vi "absolute_position.vi"(6 "ENCODER rotates cw":bool, 7 "curr. angle":dbl format="%#_13g", 8 "Absolute position in":dbl=-1.0, 11 "prev. angle":dbl format="%#_13g") -> (0 "Absolute position out":dbl, 1 "relative position Gantry":dbl, 2 "relative position shaft":dbl, 3 "Gantry Position (abs)":dbl)   [LabVIEW 2021]
panel:
  out "abs(x)":dbl
  out "angular step > 8deg and <345?":bool
  out "angular difference":dbl
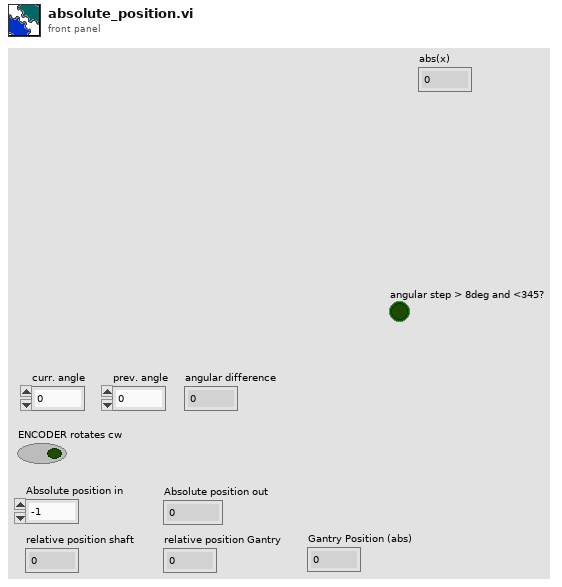
[diagram p1: front panel]
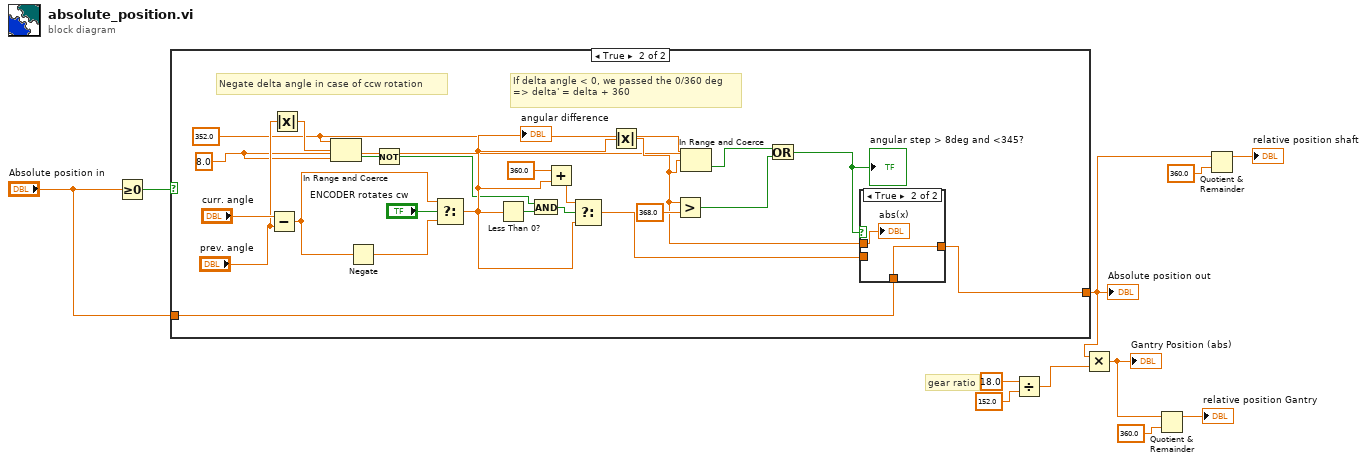
[diagram p0: block diagram]
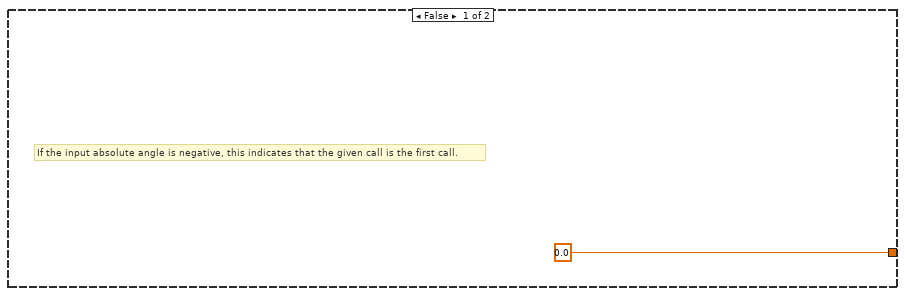
[diagram p2: hidden frame]
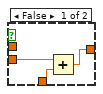
[diagram p3: hidden frame]
diagram:
  # "gear ratio"
  n1 = Greater Or Equal To 0?(x="Absolute position in") -> (x >= 0?=w8:bool)
  n2 = case shown="True" w8 {
    tunnel: "Absolute position in" -> [_ w29]
    tunnel: [0.0 w27] -> w5
    frame False {
      # "If the input absolute angle is negative, this indicates that the given call is the first call."
    }
    frame True {
      w18 = 352.0 ("upper limit")
      w17 = 8.0 ("y")
      # "If delta angle < 0, we passed the 0/360 deg => delta' = delta + 360"
      # "Negate delta angle in case of ccw rotation"
      n3 = Subtract(x="curr. angle", y="prev. angle") -> (x-y=w31:dbl)
      n4 = Absolute Value(x="prev. angle") -> (abs(x)=w19:dbl)
      n5 = In Range and Coerce(upper limit=w18, x=w19, lower limit=w17) -> (In Range?=w16:bool)  [unwired: 1 out]
      n6 = Negate(x=w31) -> (-x=w30:dbl)
      n7 = Not(x=w16) -> (.not. x?=w14:bool)
      n8 = Select(t=w31, s="ENCODER rotates cw", f=w30) -> (s? t:f=w26:dbl)
      "angular difference" <- w26
      n9 = Less Than 0?(x=w26) -> (x < 0?=w15:bool)
      n10 = And(x=w14, y=w15) -> (x .and. y?=w13:bool)
      n11 = Add(x=360.0, y=w26) -> (x+y=w32:dbl)
      n12 = Select(t=w32, s=w13, f=w26) -> (s? t:f=w28:dbl)
      n13 = Absolute Value(x=w26) -> (abs(x)=w21:dbl)
      n14 = Greater?(x=w21, y=368.0) -> (0:w23:bool)
      n15 = In Range and Coerce(upper limit=w18, x=w21, lower limit=w17) -> (In Range?=w25:bool)  [unwired: 1 out]
      n16 = Or(x=w25, y=w23) -> (x .or. y?=w22:bool)
      "angular step > 8deg and <345?" <- w22
      n17 = case shown="True" w22 {
        tunnel: w29 -> [w38 w40]
        tunnel: w28 -> [w37 _]
        tunnel: [w36 w40] -> w27
        tunnel: w21 -> [_ w39]
        frame False {
          n18 = Add(x=w37, y=w38) -> (x+y=w36:dbl)
        }
        frame True {
          "abs(x)" <- w39
        }
      }
    }
  }
  "Absolute position out" <- w5
  n19 = Divide(x=18.0, y=152.0) -> (x/y=w9:dbl)
  n20 = Multiply(x=w5, y=w9) -> (x*y=w1:dbl)
  "Gantry Position (abs)" <- w1
  n21 = Quotient & Remainder(x=w1, y=360.0) -> (x-y*floor(x/y)=→"relative position Gantry":dbl)  [unwired: 1 out]
  n22 = Quotient & Remainder(x=w5, y=360.0) -> (x-y*floor(x/y)=→"relative position shaft":dbl)  [unwired: 1 out]
